vi "Wait Data.vi"(8 "error in (no error)":errorcluster, 11 "Event in":refnum<class "Event.lvclass">) -> (0 "error out":errorcluster, 1 "Timeout Occurred":bool=TRUE, 2 "Data out":refnum<class "Data.lvclass">, 3 "Event out":refnum<class "Event.lvclass">)   [LabVIEW 2015, in "MDSplus.lvlib" / "Event.lvclass"]
doc: "Return data received last."
uses:
  <vilib>/MDSplus/Classes/Event_Class/Event.lvclass
  <vilib>/MDSplus/Classes/Data_Class/Data.lvclass
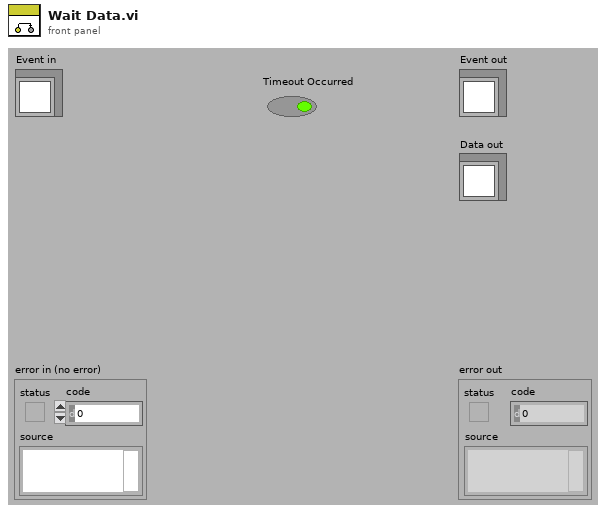
[diagram p1: front panel]
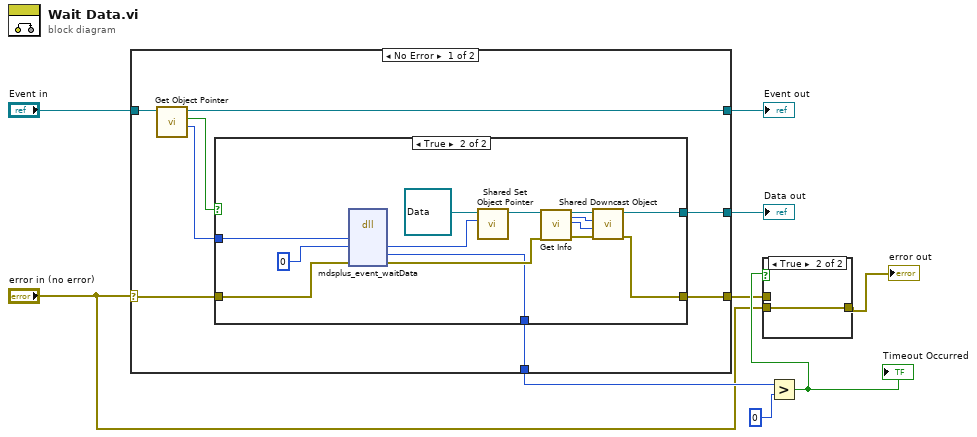
[diagram p0: block diagram]
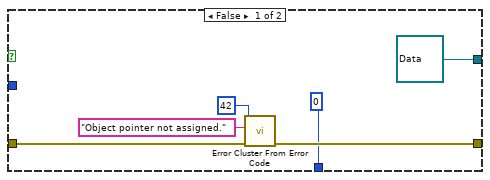
[diagram p3: hidden frame]
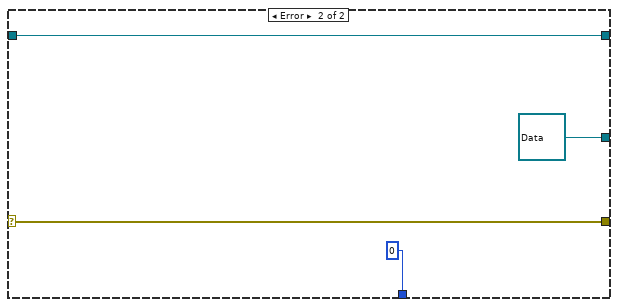
[diagram p4: hidden frame]
diagram:
  n1 = case shown="No Error" "error in (no error)" {
    selector: "error in (no error)" -> [w13 w41]
    tunnel: [w12 w41] -> w1
    tunnel: [w11 w40] -> w8
    tunnel: "Event in" -> [w16 w40]
    tunnel: [w17 refnum<class "Data.lvclass"> refnum ("Data out")] -> w7
    tunnel: [w10 0] -> w6
    frame No Error {
      n2 = call-dynamic "Get Object Pointer.vi"("Event in"=w16) -> ("Object Pointer"=w14:i64, "Assigned object pointer?"=w15:bool, "Event out"=w11:refnum<class "Event.lvclass">)  [unwired: 8 in]
      n3 = case shown="True" w15 {
        tunnel: [refnum<class "Data.lvclass"> refnum ("Data out") w29] -> w17
        tunnel: w14 -> [_ w28]
        tunnel: w13 -> [w20 w26]
        tunnel: [w19 w25] -> w12
        tunnel: [0 w24] -> w10
        frame False {
          n4 = call <vilib>:"Error Cluster From Error Code.vi"("error in (no error)"=w20, "error message (\"\")"="Object pointer not assigned." ("error message (\"\")"), "error code (0)"=42) -> ("error out"=w19:errorcluster)  [unwired: 6 in]
        }
        frame True {
          n5 = dll-call lib="MDSobjectsLVShr" fn="mdsplus_event_waitData"("lvEventPtr"=w28, "lvDataPtrOut"=i64 0, "error"=w26) -> ("lvDataPtrOut"=w35:i64, "timeoutOccurred"=w24:i32, "error"=w27:errorcluster)  [unwired: 6 in, 2 out]
          n6 = call <vilib>:"Shared Set Object Pointer.vi"("Object Pointer"=w35, "Data in"=refnum<class "Data.lvclass"> refnum ("Data.lvclass")) -> ("Data out"=w34:refnum<class "Data.lvclass">)  [unwired: 9 in]
          n7 = call-dynamic "Get Info.vi"("Data in"=w34, "error in (no error)"=w27) -> ("Data out"=w33:refnum<class "Data.lvclass">, "Class type out"=w32:u8, "Data type out"=w31:u8, "error out"=w30:errorcluster)  [unwired: 12 in, 2 out]
          n8 = call <vilib>:"Shared Downcast Object.vi"("error in (no error)"=w30, "Data Type"=w31, "Class Type"=w32, "Data in"=w33) -> ("error out"=w25:errorcluster, "Data out"=w29:refnum<class "Data.lvclass">)  [unwired: 6 in]
        }
      }
    }
    frame Error {
    }
  }
  "Event out" <- w8
  "Data out" <- w7
  n9 = Greater?(x=w6, y=0) -> (0:w4:bool)
  "Timeout Occurred" <- w4
  n10 = case shown="True" w4 {
    tunnel: "error in (no error)" -> [_ w43]
    tunnel: [w42 w43] -> w2
    tunnel: w1 -> [w42 _]
    frame False {
    }
    frame True {
    }
  }
  "error out" <- w2
